vi "satellite simulator control.vi"() -> ()   [LabVIEW 2012]
uses:
  <vilib>/Utility/error.llb/DialogType.ctl
  <vilib>/DAQmx/create/channels.llb/DAQmx Create Channel (DO-Digital Output).vi
  <vilib>/Instr/_visa.llb/VISA Configure Serial Port (Instr).vi
  <vilib>/vision/NI_Vision_Development_Module.lvlib
  <vilib>/ptbypt/NI_PtbyPt.lvlib
panel:
  in  "Reaction Wheel":bool
  out "Write String":string
  in  "Control Value":sgl=1.5 format="%.4f"
  in  "Control Mode":u16(ring) items=["Idle"=0, "PWM (-1..1)"=1, "Current (-2.5..2.5A)"=2, "Speed (Rads/s)"=3, "Acceleration (Rads/sec^2)"=16, "Momentum (N-m-sec)"=17, "Torque (N-m)"=18]
  in  "Address":i32=11
  in  "Dst":i32=36
  in  "stop bits":u16(ring)=10 items=["1.0"=10, "1.5"=15, "2.0"=20]
  in  "VISA resource name (write)":refnum<visa-resource-name>="COM4"
  in  "flow control":u16(ring) items=["None"=0, "XON/XOFF"=1, "RTS/CTS"=2, "DTR/DSR"=4]
  in  "parity (0:none)":u16(ring) items=["None", "Odd", "Even", "Mark", "Space"]
  in  "data bits (8)":u16=8 min=5 max=8 step=1
  in  "baud rate (115200)":u32=115200
  out "bytes written":u32
  in  "bytes to read":u32=5
  out "Read string":string
  out "bytes read":u32
  out "Filtered Ohmega":dbl format="%0.2f"
  in  "VISA resource name":refnum<visa-resource-name>
  out "read buffer":string
  out "Ohmega":dbl[](graph)
  out "Filtered Ohmega":dbl[](graph)
  in  "Floating":bool
  in  "Thruster 8":bool
  in  "Thruster 7":bool
  in  "Thruster 6":bool
  in  "Thruster 5":bool
  in  "Thruster 4":bool
  in  "Thruster 3":bool
  in  "Thruster 2":bool
  in  "Truster1":bool
  in  "Thrusters Bundled":bool=TRUE
  in  "Manual Control Mode (Default)":bool
  in  "Up":bool
  in  "Right":bool
  in  "Down":bool
  in  "Left":bool
  in  "Stop 2":bool
  in  "CntrClk":bool
  in  "ClkWise":bool
  in  "Angular Acceleration":u16(ring) items=["Fast", "Slow"]
  in  "Duty Cycle":dbl=1.0
  in  "Automatic PD Position Controller":bool
  in  "Pixel-Distance Ratio (pix/cm)":dbl=8.26
  in  "Remote Logger Status":bool
  in  "Downlink Object Data?":bool
  in  "Remote Port":u16=61557
  in  "Local Port":u16=61556
  in  "Remote Host":string="localhost"
  in  "broadcast":bool
  in  "Maintain Attitude":bool
  out "alpha":dbl
  out "Objects":T1(array[cluster]) {"Aspect Ratio" format="%.2f"; "Orientation" format="%.2f"; "Area" format="%.2f"; "Object Center"."Y" format="%.2f"; "Object Center"."X" format="%.2f"}
  in  "Y Center Correction":dbl
  in  "X Center Correction":dbl
  out "Offset Degree":dbl
  in  "Y Desired":dbl
  in  "X Desired":dbl
  out "Vx (cm/s)":dbl
  out "Vy (cm/s)":dbl
  in  "OK Button":bool
  in  "Air Floating Status":bool
  in  "Control Freq":u32=20
  in  "Alpha Desired":dbl
  in  "STOP":bool caption="stop (F)"
  out "Image Out":T2(plugin-control)
  out "alpha (deg)":dbl
  out "dx (cm)":dbl
  out "dy (cm)":dbl
  # "Bundled Operations"
  # "Unbundled Operations"
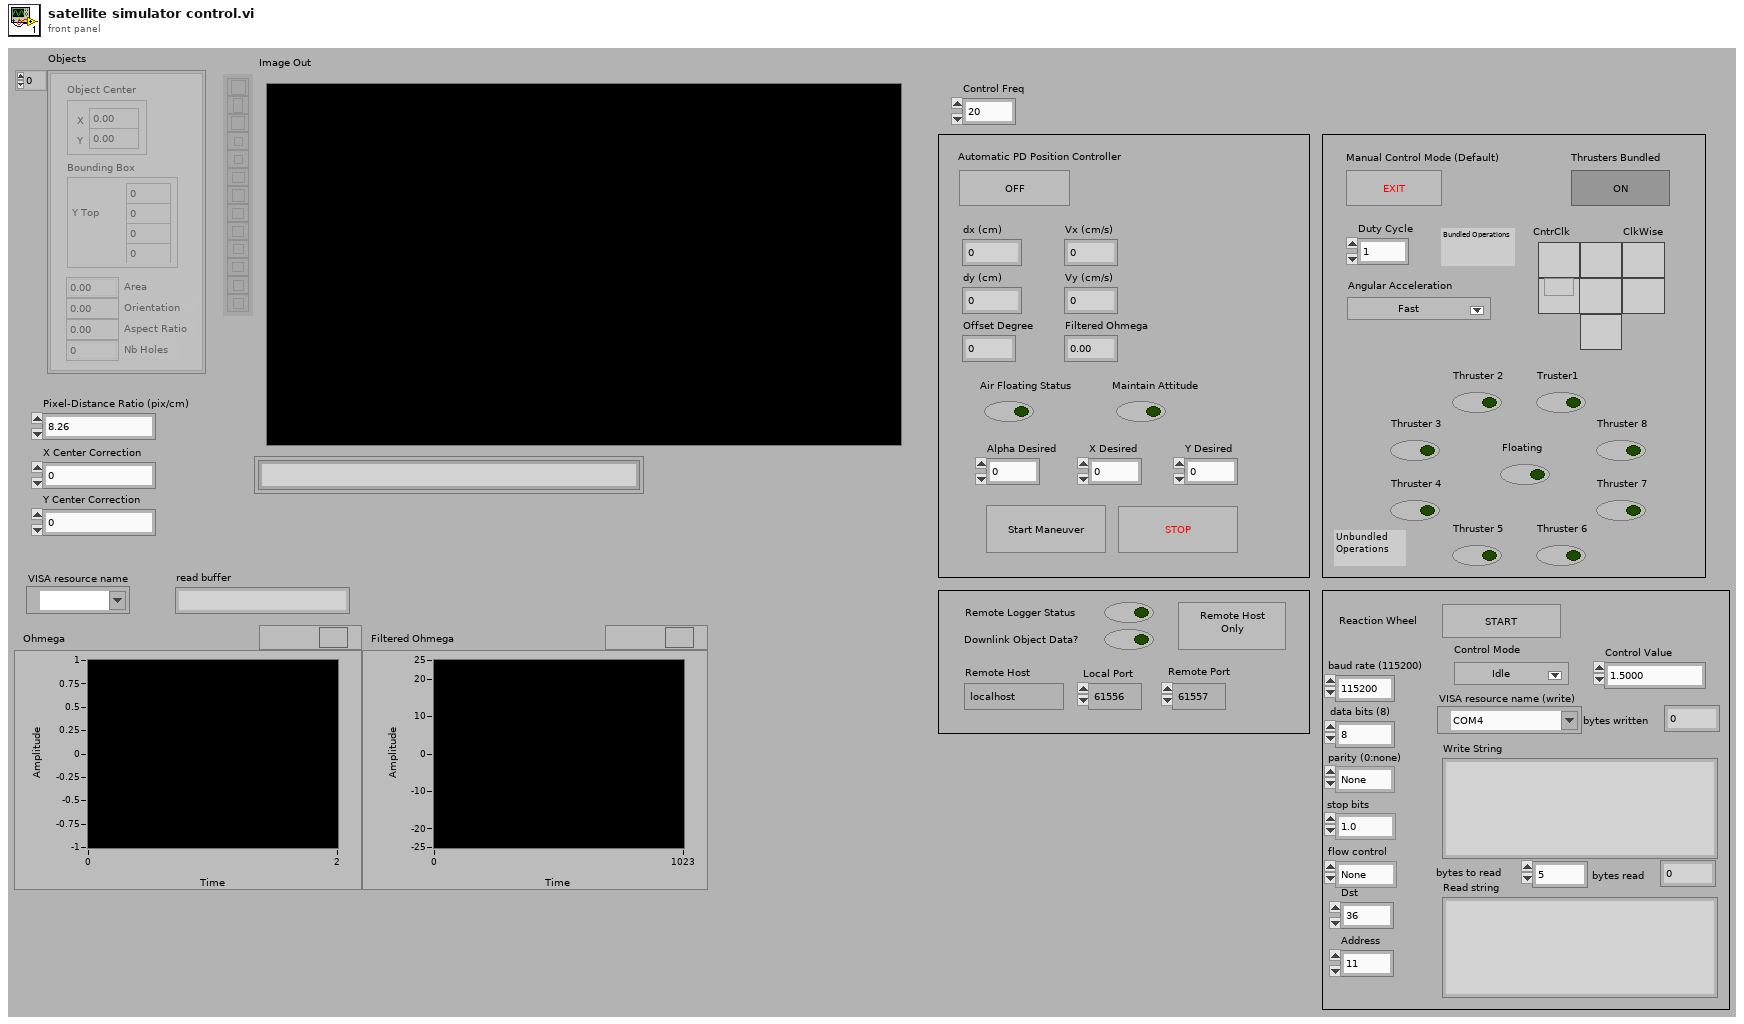
[diagram p1: front panel]
types:
  T1 = cluster{"Object Center":cluster{"X":sgl, "Y":sgl}, "Bounding Box":cluster{"X Left":i32, "Y Top":i32, "X Right":i32, "Y Bottom":i32}, "Area":sgl, "Orientation":sgl, "Aspect Ratio":sgl, "Nb Holes":i32}[]
  T2 = typedef "IMAQ Image.ctl" = refnum<image>
  T3 = typedef "DialogType.ctl" = u16
  T4 = cluster{"dx (cm)":dbl, "dy (cm)":dbl, "Offset Degree":dbl}
  T5 = cluster{"Objects":u16, "Threshold":i32, "Reject Border":bool, "Fill Holes":bool, "Min Object Size":bool, "Min Size":i32, "Max Object Size":bool, "Max Size":i32, "Show Search Area":bool, "Show Center":bool, "Show Bounding Box":bool}
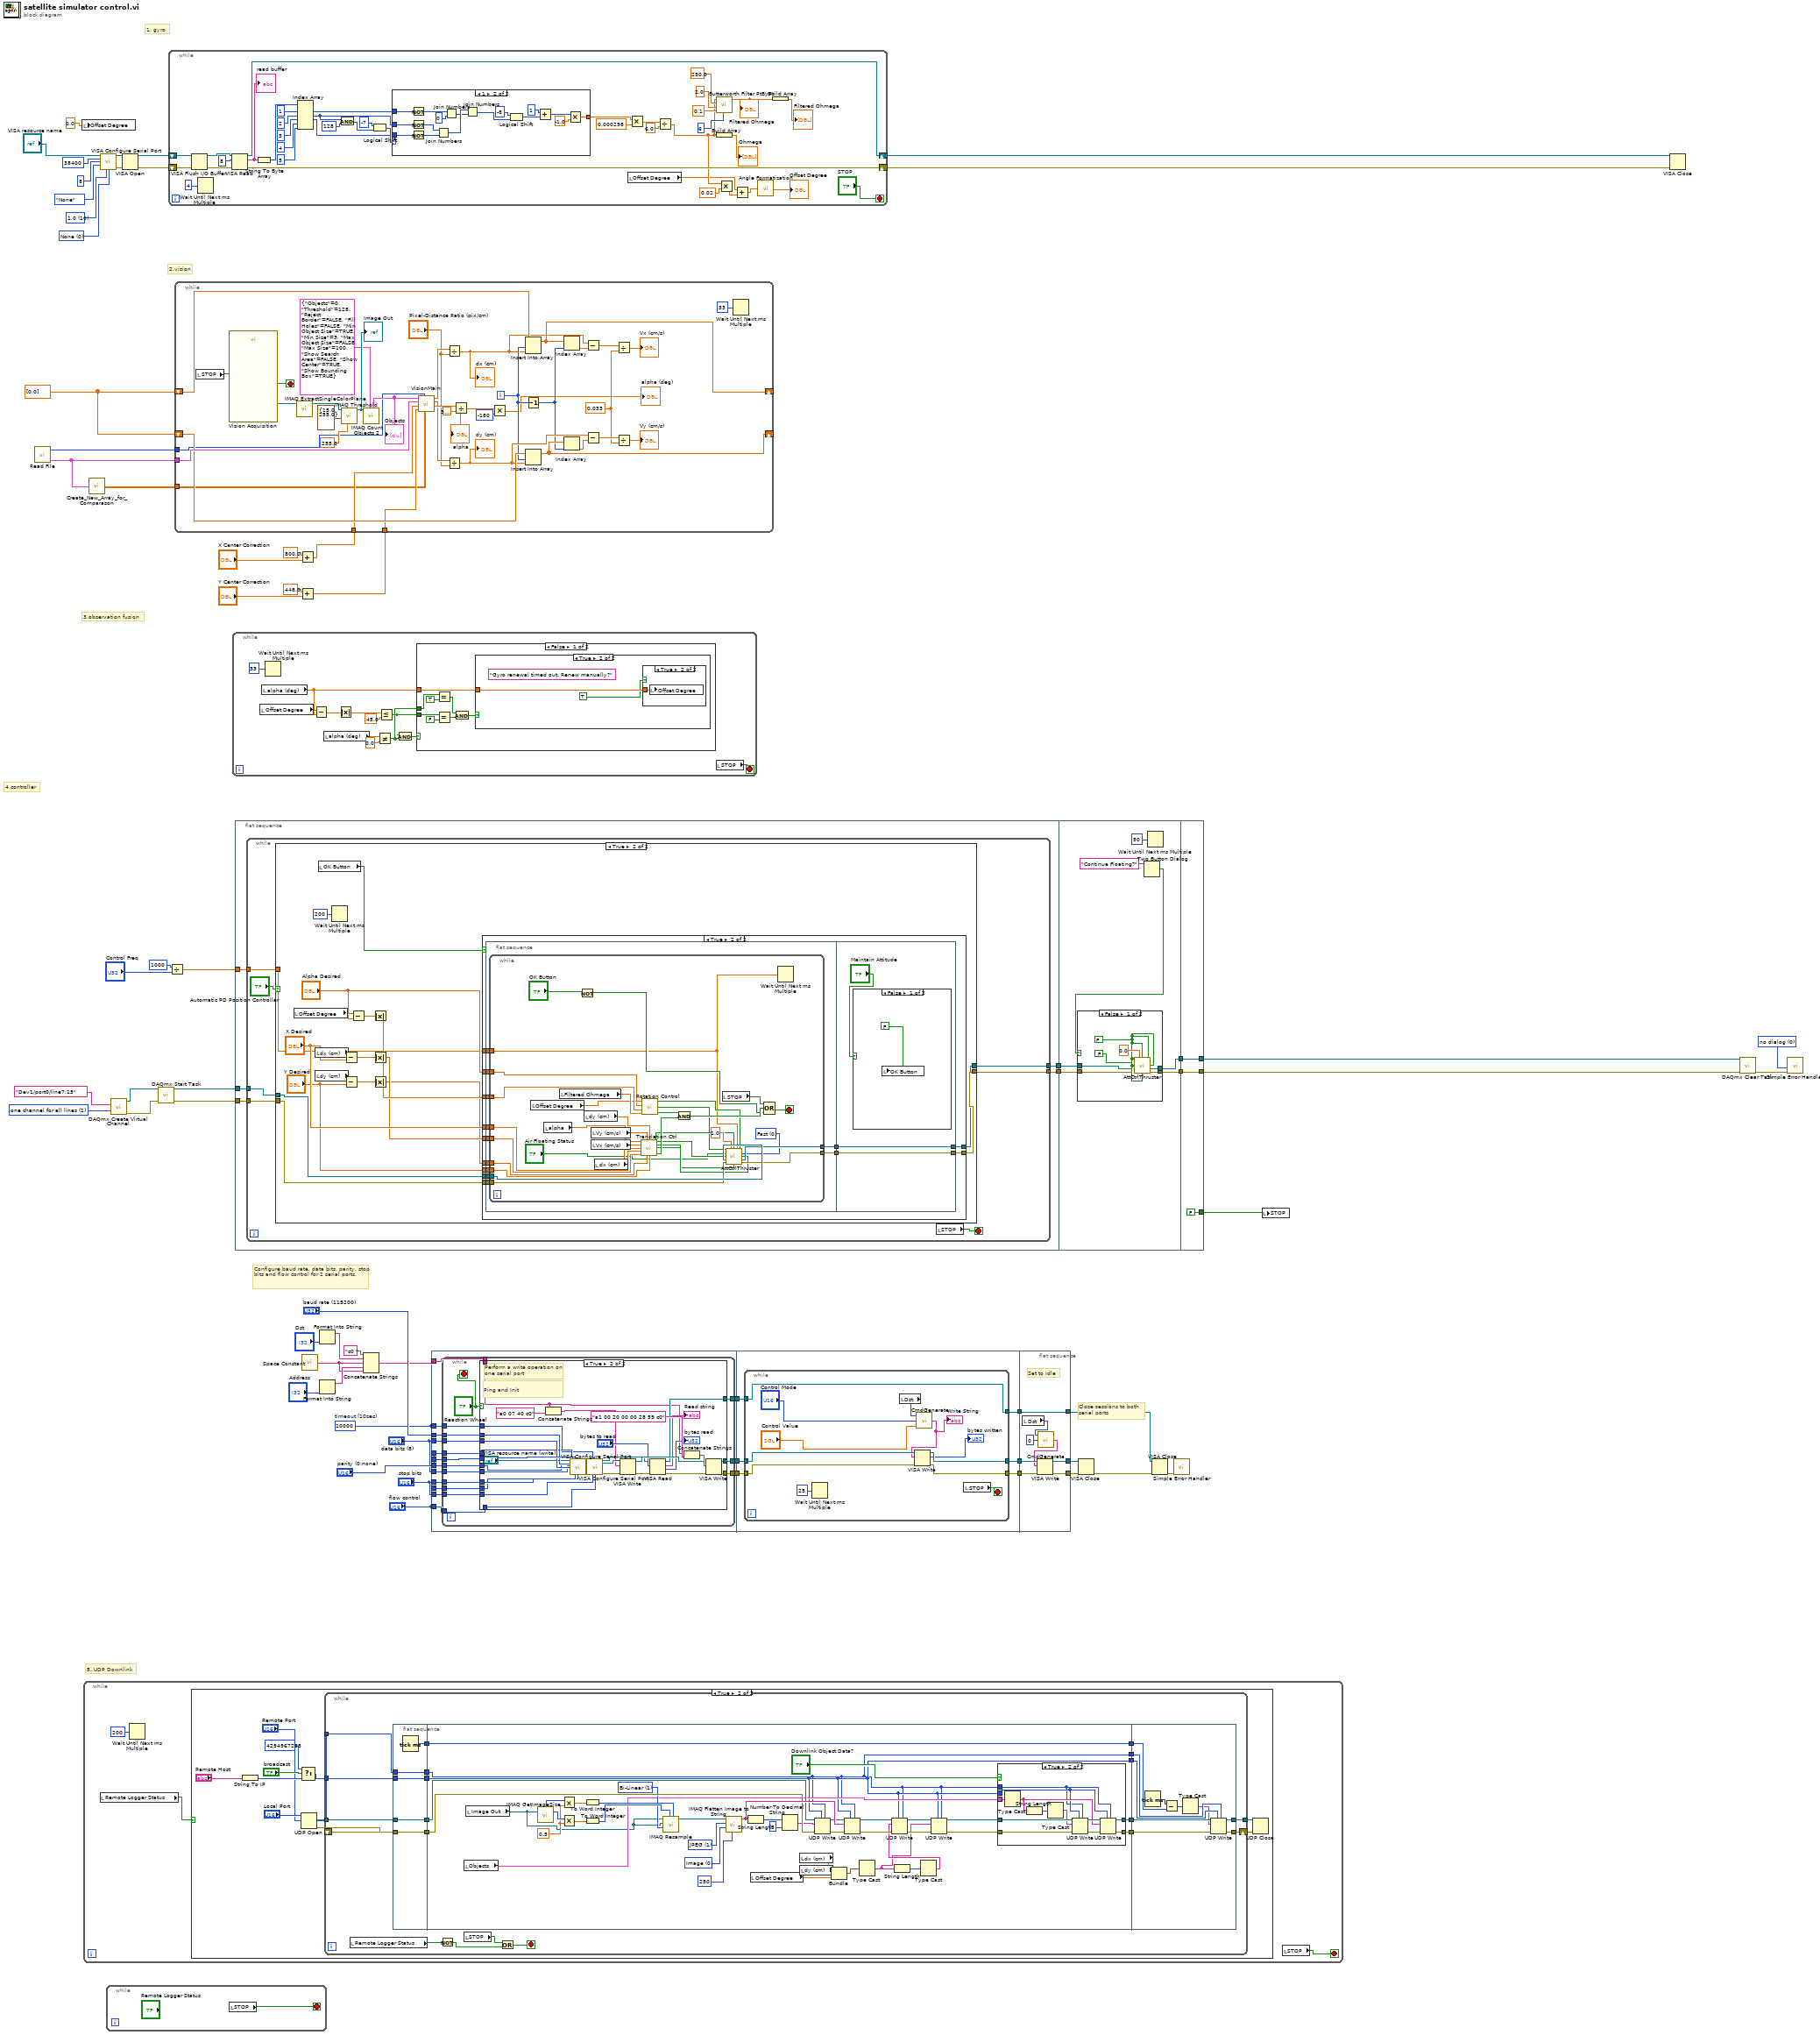
[diagram p0: block diagram]
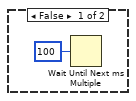
[diagram p2: hidden frame]
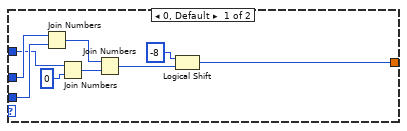
[diagram p3: hidden frame]
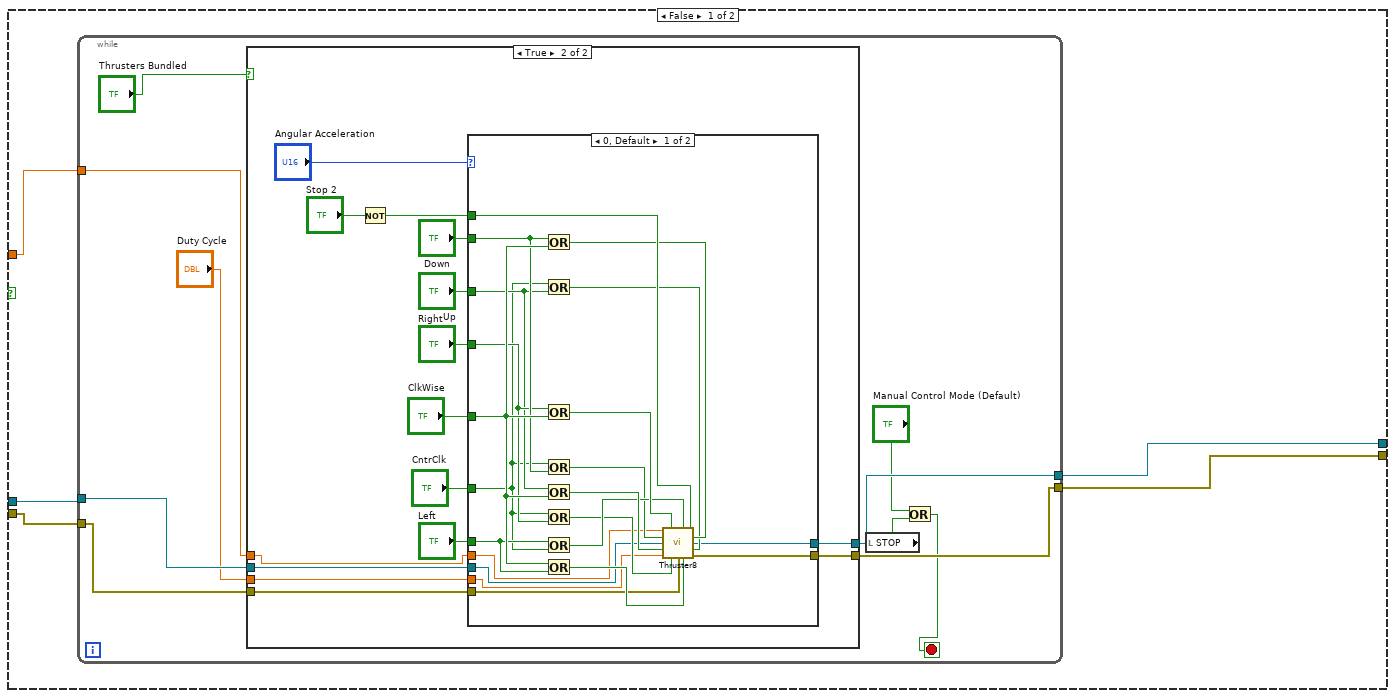
[diagram p6: hidden frame]
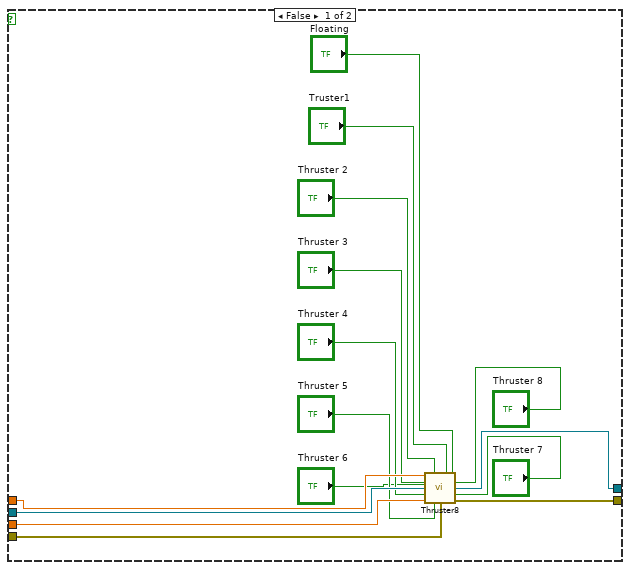
[diagram p7: hidden frame]
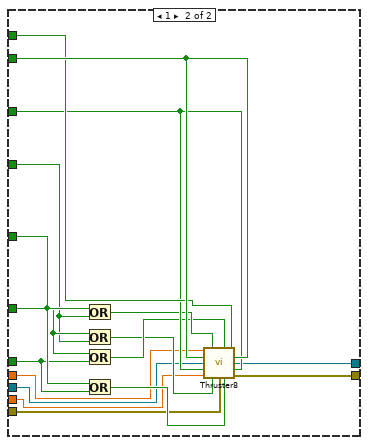
[diagram p8: hidden frame]
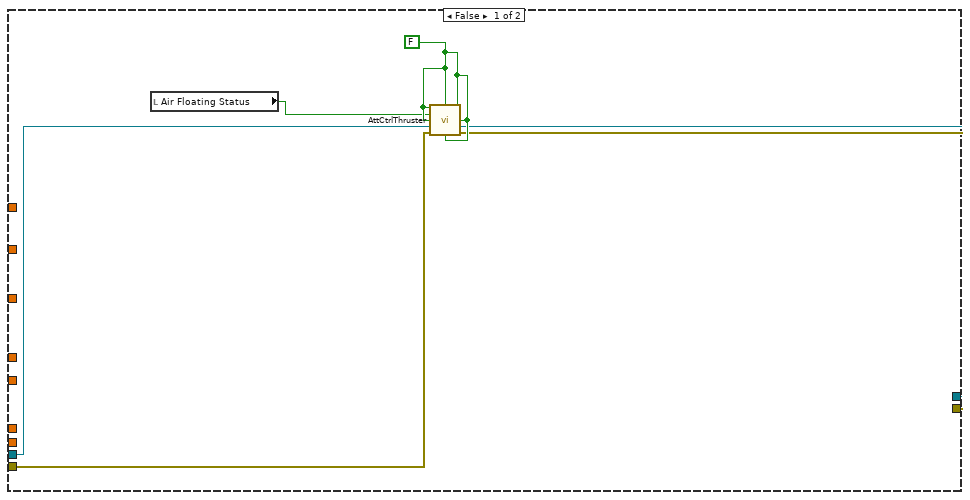
[diagram p9: hidden frame]
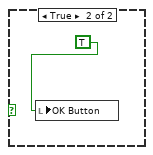
[diagram p10: hidden frame]
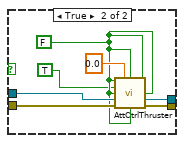
[diagram p11: hidden frame]
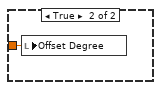
[diagram p14: hidden frame]
diagram:
  w11 = u32 10000  # timeout (10sec)
  w28 = u16 0 items=["None", "XON/XOFF", "RTS/CTS", "XON/XOFF & RTS/CTS", "DTR/DSR", "XON/XOFF & DTR/DSR"] ("flow control (0:none)")
  w30 = u16 10 items=["1.0"=10, "1.5"=15, "2.0"=20] ("stop bits (10: 1 bit)")
  w60 = T3 0 items=["no dialog", "OK message", "continue or stop message", "OK message + warnings", "continue/stop + warnings"] ("type of dialog (OK msg:1)")
  w63 = 1 items=["one channel for each line", "one channel for all lines"] ("line grouping")
  w49 = dbl[] [0.0]
  # "Close sessions to both serial ports"
  # "Configure baud rate, data bits, parity, stop bits and flow control for 2 serial ports."
  # "5. UDP Downlink"
  # "4.controller"
  # "3.observation fusion"
  # "2.vision"
  # "1. gyro"
  n1 = call "Read File.vi"() -> ("Objects"=w27:T1, "Total Obj"=w25:i32)  [unwired: 1 in]
  n2 = local write "Offset Degree"(0.0 ("y")) -> ()
  n3 = while {
    stop <- w67 stop-if-true
    n4 = local read "Remote Logger Status"() -> (w68:bool)
    n5 = Wait Until Next ms Multiple(millisecond multiple=u32 200) -> ()  [unwired: 1 out]
    n6 = case shown="True" w68 {
      frame False {
      }
      frame True {
        n7 = String To IP(1:"Remote Host") -> (0:w76:u32)
        n8 = Select(t=u32 4294967295, s="broadcast", f=w76) -> (s? t:f=w73:u32)
        n9 = UDP Open(11:"Local Port") -> (port=w72:refnum<k16>, 0:w71:errorcluster)  [unwired: 1 in, 4 out]
        n10 = while {
          tunnel: "Remote Port" -> [w99]
          tunnel: w73 -> [w98]
          tunnel: w72 -> [w97]
          tunnel: [w95] -> w70
          shift-right: [w94] -> w69
          shift-left: w71 -> [w96]
          stop <- w83 stop-if-true
          n11 = local read "Remote Logger Status"() -> (w81:bool)
          n12 = flat-sequence {
            tunnel: w97 -> [w101]
            tunnel: w99 -> [w102]
            tunnel: w98 -> [w103]
            tunnel: w96 -> [w104]
            tunnel: [w104] -> w93
            tunnel: [w103] -> w92
            tunnel: [w102] -> w91
            tunnel: [w101] -> w90
            tunnel: [w100] -> w89
            tunnel: [w124] -> w88
            tunnel: [w123] -> w87
            tunnel: w93 -> [w142]
            tunnel: w92 -> [w106]
            tunnel: w91 -> [w105]
            tunnel: w90 -> [w126]
            tunnel: [w125] -> w86
            tunnel: w89 -> [w125]
            tunnel: [w105] -> w85
            tunnel: [w106] -> w84
            tunnel: [w166] -> w95
            tunnel: [w160] -> w94
            tunnel: w88 -> [w161]
            tunnel: w87 -> [w167]
            tunnel: w86 -> [w168]
            tunnel: w85 -> [w165]
            tunnel: w84 -> [w164]
            frame #0 {
              n13 = Tick Count (ms)() -> (millisecond timer value=w100:u32)
            }
            frame #1 {
              w130 = u32 1 items=["Zero Order", "Bi-Linear", "Quadratic", "Cubic Spline"] ("Interpolation Type")
              w131 = 0.5
              w139 = 0 items=["Image", "Image and Vision Info", "Reference to Image"] ("Type of Flatten (Image and Vision Info)")
              w144 = 1 items=["None", "JPEG", "PACKED BINARY"] ("Compression (None)")
              n14 = local read "Objects"() -> (w121:T1)
              n15 = local read "Image Out"() -> (w120:T2)
              n16 = call "IMAQ GetImageSize"("Image"=w120) -> ("Y Resolution"=w132:i32, "X Resolution"=w133:i32)  [unwired: 3 in, 1 out]
              n17 = Multiply(x=w133, y=w131) -> (x*y=w135:dbl)
              n18 = Multiply(x=w132, y=w131) -> (x*y=w137:dbl)
              n19 = To Word Integer(number=w135) -> (16bit integer=w134:i16)
              n20 = To Word Integer(number=w137) -> (16bit integer=w136:i16)
              n21 = call "IMAQ Resample"("X Resolution"=w134, "Y Resolution"=w136, "Interpolation Type"=w130, "Image Dst"=w120, "Image Src"=w120) -> ("Image Dst Out"=w138:T2)  [unwired: 5 in, 1 out]
              n22 = call "IMAQ Flatten Image to String"("Quality (750)"=250, "Type of Flatten (Image and Vision Info)"=w139, "Compression (None)"=w144, "Image"=w138) -> ("Data String"=w143:string)  [unwired: 6 in, 1 out]
              n23 = String Length(string=w143) -> (length=w129:i32)
              n24 = local read "Offset Degree"() -> (w117:dbl)
              n25 = Number To Decimal String(number=w129, width (-)=i16 5) -> (decimal integer string=w128:string)
              n26 = local read "dx (cm)"() -> (w119:dbl)
              n27 = local read "dy (cm)"() -> (w118:dbl)
              n28 = UDP Write(address=w106, port or service name=w105, connection ID=w126, data in=w128, 8:w142) -> (error out=w141:errorcluster, 3:w140:refnum<k16>)  [unwired: 1 out]
              n29 = Bundle("dx (cm)"=w119, "dy (cm)"=w118, "Offset Degree"=w117) -> (w116:T4)  [unwired: 1 in]
              n30 = UDP Write(address=w106, port or service name=w105, connection ID=w140, data in=w143, 8:w141) -> (error out=w114:errorcluster, 3:w115:refnum<k16>)  [unwired: 1 out]
              n31 = Type Cast(x=w116) -> (*(type *) &x=w107:string)  [unwired: 1 in]
              n32 = String Length(string=w107) -> (length=w109:i32)
              n33 = Type Cast(x=w109) -> (*(type *) &x=w108:string)  [unwired: 1 in]
              n34 = UDP Write(address=w106, port or service name=w105, connection ID=w115, data in=w108, 8:w114) -> (error out=w113:errorcluster, 3:w111:refnum<k16>)  [unwired: 1 out]
              n35 = UDP Write(address=w106, port or service name=w105, connection ID=w111, data in=w107, 8:w113) -> (error out=w112:errorcluster, 3:w110:refnum<k16>)  [unwired: 1 out]
              n36 = case shown="True" "Downlink Object Data?" {
                tunnel: w121 -> [_ w159]
                tunnel: w112 -> [w147 w157]
                tunnel: [w147 w155] -> w124
                tunnel: w110 -> [w146 w154]
                tunnel: [w146 w152] -> w123
                tunnel: w106 -> [_ w149]
                tunnel: w105 -> [_ w148]
                frame False {
                }
                frame True {
                  n37 = Type Cast(x=w159) -> (*(type *) &x=w150:string)  [unwired: 1 in]
                  n38 = String Length(string=w150) -> (length=w158:i32)
                  n39 = Type Cast(x=w158) -> (*(type *) &x=w151:string)  [unwired: 1 in]
                  n40 = UDP Write(address=w149, port or service name=w148, connection ID=w154, data in=w151, 8:w157) -> (error out=w156:errorcluster, 3:w153:refnum<k16>)  [unwired: 1 out]
                  n41 = UDP Write(address=w149, port or service name=w148, connection ID=w153, data in=w150, 8:w156) -> (error out=w155:errorcluster, 3:w152:refnum<k16>)  [unwired: 1 out]
                }
              }
            }
            frame #2 {
              n42 = Tick Count (ms)() -> (millisecond timer value=w169:u32)
              n43 = Subtract(x=w169, y=w168) -> (x-y=w163:u32)
              n44 = Type Cast(x=w163) -> (*(type *) &x=w162:string)  [unwired: 1 in]
              n45 = UDP Write(address=w164, port or service name=w165, connection ID=w167, data in=w162, 8:w161) -> (error out=w160:errorcluster, 3:w166:refnum<k16>)  [unwired: 1 out]
            }
          }
          n46 = Not(x=w81) -> (.not. x?=w80:bool)
          n47 = local read "STOP"() -> (w82:bool)
          n48 = Or(x=w82, y=w80) -> (x .or. y?=w83:bool)
        }
        n49 = UDP Close(connection ID=w70, 8:w69) -> ()  [unwired: 2 out]
      }
    }
    n50 = local read "STOP"() -> (w67:bool)
  }
  n51 = call "Create_New_Array_for_Comparason.vi"("Captured Plots"=w27) -> ("Generated Distance Array"=w26:dbl[][])
  n52 = call-poly "VISA Configure Serial Port"("VISA resource name"="VISA resource name", "baud rate (9600)"=u32 38400, "data bits (8)"=u16 8, "parity (0:none)"=enum16{"None", "Odd", "Even", "Mark", "Space"}."None", "stop bits (10: 1 bit)"=w30, "flow control (0:none)"=w28) -> ("VISA resource name out"=w37:refnum<visa-resource-name>, "error out"=w36:errorcluster)  [unwired: 8 in]
  n53 = while {
    stop <- w170 stop-if-true
    n54 = local read "STOP"() -> (w170:bool)
  }
  n55 = call-poly <vilib>:"DAQmx Create Virtual Channel.vi"("lines"=tag "Dev1/port0/line7:15" ("Lines"), "line grouping"=w63) -> ("task out"=w61:refnum<k21>, "error out"=w62:errorcluster)  [unwired: 12 in]
  n56 = VISA Open(error in (no error)=w36, VISA resource name=w37) -> (VISA resource name=w35:refnum<visa-resource-name>, error out=w34:errorcluster)  [unwired: 3 in]
  n57 = call <vilib>:"DAQmx Start Task.vi"("task/channels in"=w61, "error in"=w62) -> ("task out"=w56:refnum<k21>, "error out"=w55:errorcluster)  [unwired: 12 in]
  n58 = while {
    shift-right: [w178] -> w32
    shift-left: w34 -> [w208]
    shift-right: [w179] -> w33
    shift-left: w35 -> [w209]
    stop <- "STOP" stop-if-true
    n59 = VISA Flush I/O Buffer(VISA resource name=w209, error in (no error)=w208) -> (VISA resource name out=w207:refnum<visa-resource-name>, error out=w206:errorcluster)  [unwired: 1 in]
    n60 = Wait Until Next ms Multiple(millisecond multiple=u32 4) -> ()  [unwired: 1 out]
    n61 = VISA Read(VISA resource name=w207, byte count=u32 8, error in (no error)=w206) -> (VISA resource name out=w179:refnum<visa-resource-name>, read buffer=w180:string, error out=w178:errorcluster)  [unwired: 1 out]
    "read buffer" <- w180
    n62 = String To Byte Array(string=w180) -> (unsigned byte array=w201:u8[])
    n63 = Index Array(array=w201, index #1=1 ("index"), index #2=2 ("index"), index #3=3 ("index"), index #4=4 ("index"), index #5=5 ("index")) -> (element #1=w185:u8, element #2=w184:u8, element #3=w183:u8)  [unwired: 2 out]
    n64 = And(x=w184, y=u8 128) -> (x .and. y?=w195:u8)
    n65 = Logical Shift(y=i16 -7, x=w195) -> (x << y=w193:u8)
    n66 = case shown="1" w193 {
      tunnel: [w211 w220] -> w197
      tunnel: w185 -> [w212 w230]
      tunnel: w184 -> [w214 w229]
      tunnel: w183 -> [w213 w228]
      frame 0, Default {
        n67 = Join Numbers(hi=w214, lo=w213) -> ((hi.lo)=w219:u16)
        n68 = Join Numbers(hi=w212, lo=u8 0) -> ((hi.lo)=w217:u16)
        n69 = Join Numbers(hi=w219, lo=w217) -> ((hi.lo)=w216:u32)
        n70 = Logical Shift(y=i16 -8, x=w216) -> (x << y=w211:u32)
      }
      frame 1 {
        n71 = Not(x=w230) -> (.not. x?=w225:u8)
        n72 = Not(x=w229) -> (.not. x?=w227:u8)
        n73 = Not(x=w228) -> (.not. x?=w226:u8)
        n74 = Join Numbers(hi=w227, lo=w226) -> ((hi.lo)=w235:u16)
        n75 = Join Numbers(hi=w225, lo=u8 0) -> ((hi.lo)=w233:u16)
        n76 = Join Numbers(hi=w235, lo=w233) -> ((hi.lo)=w232:u32)
        n77 = Logical Shift(y=i16 -8, x=w232) -> (x << y=w224:u32)
        n78 = Add(x=u32 1, y=w224) -> (x+y=w221:u32)
        n79 = Multiply(x=w221, y=-1.0) -> (x*y=w220:dbl)
      }
    }
    n80 = local read "Offset Degree"() -> (w174:dbl)
    n81 = Multiply(x=w197, y=0.000298) -> (x*y=w203:dbl)
    n82 = Divide(x=w203, y=6.0) -> (x/y=w175:dbl)
    n83 = call <vilib>:"Butterworth Filter PtByPt.vi"("order"=6, "low cutoff freq: fl"=0.1, "high cutoff freq: fh"=2.0, "sampling freq: fs"=250.0, "x"=w175) -> ("Filtered x"=w187:dbl)  [unwired: 4 in, 1 out]
    "Filtered Ohmega" <- w187
    n84 = Build Array(w175) -> (→"Ohmega":dbl[])
    n85 = Multiply(x=w175, y=0.02) -> (x*y=w173:dbl)
    n86 = Add(x=w174, y=w173) -> (x+y=w172:dbl)
    n87 = call "Angle Formatization.vi"("Alpha"=w172) -> ("Alpha Formatized"=→"Offset Degree":dbl)
    n88 = Build Array(w187) -> (→"Filtered Ohmega":dbl[])
  }
  n89 = Divide(x=u32 1000 ("milliseconds to wait"), y="Control Freq") -> (x/y=w52:dbl)
  n90 = while {
    stop <- w246 stop-if-true
    n91 = local read "Offset Degree"() -> (w245:dbl)
    n92 = local read "alpha (deg)"() -> (w241:dbl)
    n93 = Wait Until Next ms Multiple(millisecond multiple=u32 33) -> ()  [unwired: 1 out]
    n94 = Subtract(x=w245, y=w241) -> (x-y=w244:dbl)
    n95 = local read "alpha (deg)"() -> (w239:dbl)
    n96 = Absolute Value(x=w244) -> (abs(x)=w243:dbl)
    n97 = Not Equal?(x=w239, y=0.0) -> (x != y?=w237:bool)
    n98 = Less Or Equal?(x=w243, y=45.0) -> (x <= y?=w236:bool)
    n99 = And(x=w236, y=w237) -> (x .and. y?=w240:bool)
    n100 = case shown="False" w240 {
      tunnel: w241 -> [w248 w259]
      tunnel: w237 -> [w250 _]
      tunnel: w236 -> [w249 _]
      frame False {
        n101 = Equal?(x=w250, y=TRUE) -> (x = y?=w254:bool)
        n102 = Equal?(x=w249, y=FALSE) -> (x = y?=w253:bool)
        n103 = And(x=w254, y=w253) -> (x .and. y?=w251:bool)
        n104 = case shown="True" w251 {
          tunnel: w248 -> [_ w257]
          frame False {
          }
          frame True {
            (unwired) "Gyro renewal timed out. Renew manually?" ("message")
            n105 = case shown="True" TRUE {
              tunnel: w257 -> [_ w258]
              frame False {
              }
              frame True {
                n106 = local write "Offset Degree"(w258) -> ()
              }
            }
          }
        }
      }
      frame True {
        n107 = local write "Offset Degree"(w259) -> ()
      }
    }
    n108 = local read "STOP"() -> (w246:bool)
  }
  n109 = flat-sequence {
    tunnel: w56 -> [w264]
    tunnel: w55 -> [w263]
    tunnel: w52 -> [w260]
    tunnel: [w262] -> w51
    tunnel: [w261] -> w50
    tunnel: w51 -> [w449]
    tunnel: w50 -> [w447]
    tunnel: [w448] -> w42
    tunnel: [w446] -> w41
    tunnel: [w465] -> w53
    tunnel: [w466] -> w54
    tunnel: w42 -> [w466]
    tunnel: w41 -> [w465]
    tunnel: [FALSE] -> w40
    frame #0 {
      n110 = while {
        tunnel: w264 -> [w271]
        tunnel: w263 -> [w270]
        tunnel: [w269] -> w262
        tunnel: [w268] -> w261
        tunnel: w260 -> [w266]
        stop <- w267 stop-if-true
        n111 = case shown="True" "Automatic PD Position Controller" {
          tunnel: w271 -> [w275 w373]
          tunnel: w270 -> [w274 w372]
          tunnel: [w272 w371] -> w269
          tunnel: [w273 w370] -> w268
          tunnel: w266 -> [w276 w356]
          frame False {
            n112 = while {
              tunnel: w276 -> [w286]
              tunnel: w275 -> [w285]
              tunnel: [w284] -> w273
              tunnel: [w283] -> w272
              tunnel: w274 -> [w282]
              stop <- w279 stop-if-true
              n113 = case shown="True" "Thrusters Bundled" {
                tunnel: w286 -> [w297 w309]
                tunnel: w285 -> [w301 w308]
                tunnel: [w298 w307] -> w284
                tunnel: [w299 w306] -> w283
                tunnel: w282 -> [w300 w305]
                tunnel: "Duty Cycle" -> [w296 w302]
                frame False {
                  n114 = call "Thruster8.vi"("period"=w297, "Thruster 2"="Thruster 2", "Truster1"="Truster1", "Floating"="Floating", "Thruster 3"="Thruster 3", "Thruster 8"="Thruster 8", "task in"=w301, "Thruster 4"="Thruster 4", "Thruster 7"="Thruster 7", "Duty Cycle"=w296, "Thruster 5"="Thruster 5", "error in"=w300, "Thruster 6"="Thruster 6") -> ("task out"=w298:refnum<k21>, "error out"=w299:errorcluster)  [unwired: 1 in]
                }
                frame True {
                  n115 = Not(x="Stop 2") -> (.not. x?=w303:bool)
                  n116 = case shown="0, Default" "Angular Acceleration" {
                    tunnel: w303 -> [w337 w353]
                    tunnel: "Down" -> [w329 w354]
                    tunnel: "Left" -> [w331 w347]
                    tunnel: "Up" -> [w325 w352]
                    tunnel: "Right" -> [w327 w345]
                    tunnel: "ClkWise" -> [w333 w351]
                    tunnel: "CntrClk" -> [w324 w348]
                    tunnel: w302 -> [w322 w343]
                    tunnel: w309 -> [w321 w342]
                    tunnel: w308 -> [w320 w338]
                    tunnel: [w319 w339] -> w307
                    tunnel: [w318 w340] -> w306
                    tunnel: w305 -> [w317 w341]
                    frame 0, Default {
                      n117 = Or(x=w329, y=w333) -> (x .or. y?=w332:bool)
                      n118 = Or(x=w324, y=w325) -> (x .or. y?=w323:bool)
                      n119 = Or(x=w327, y=w333) -> (x .or. y?=w335:bool)
                      n120 = Or(x=w324, y=w329) -> (x .or. y?=w328:bool)
                      n121 = Or(x=w325, y=w333) -> (x .or. y?=w336:bool)
                      n122 = Or(x=w324, y=w327) -> (x .or. y?=w326:bool)
                      n123 = Or(x=w331, y=w324) -> (x .or. y?=w330:bool)
                      n124 = Or(x=w333, y=w331) -> (x .or. y?=w334:bool)
                      n125 = call "Thruster8.vi"("period"=w321, "Thruster 2"=w335, "Truster1"=w330, "Floating"=w337, "Thruster 3"=w328, "Thruster 8"=w332, "task in"=w320, "Thruster 4"=w336, "Thruster 7"=w323, "Duty Cycle"=w322, "Thruster 5"=w326, "error in"=w317, "Thruster 6"=w334) -> ("task out"=w319:refnum<k21>, "error out"=w318:errorcluster)  [unwired: 1 in]
                    }
                    frame 1 {
                      n126 = Or(x=w351, y=w345) -> (x .or. y?=w350:bool)
                      n127 = Or(x=w348, y=w345) -> (x .or. y?=w344:bool)
                      n128 = Or(x=w348, y=w347) -> (x .or. y?=w346:bool)
                      n129 = Or(x=w351, y=w347) -> (x .or. y?=w349:bool)
                      n130 = call "Thruster8.vi"("period"=w342, "Thruster 2"=w350, "Truster1"=w346, "Floating"=w353, "Thruster 3"=w354, "Thruster 8"=w354, "task in"=w338, "Thruster 4"=w352, "Thruster 7"=w352, "Duty Cycle"=w343, "Thruster 5"=w344, "error in"=w341, "Thruster 6"=w349) -> ("task out"=w339:refnum<k21>, "error out"=w340:errorcluster)  [unwired: 1 in]
                    }
                  }
                }
              }
              n131 = local read "STOP"() -> (w281:bool)
              n132 = Or(x="Manual Control Mode (Default)", y=w281) -> (x .or. y?=w279:bool)
            }
          }
          frame True {
            n133 = local read "Offset Degree"() -> (w369:dbl)
            n134 = local read "dx (cm)"() -> (w365:dbl)
            n135 = local read "dy (cm)"() -> (w361:dbl)
            n136 = local read "OK Button"() -> (w357:bool)
            n137 = Wait Until Next ms Multiple(millisecond multiple=u32 200) -> ()  [unwired: 1 out]
            n138 = Subtract(x=w365, y="X Desired") -> (x-y=w363:dbl)
            n139 = Subtract(x=w361, y="Y Desired") -> (x-y=w359:dbl)
            n140 = Subtract(x=w369, y="Alpha Desired") -> (x-y=w367:dbl)
            n141 = Absolute Value(x=w367) -> (abs(x)=w366:dbl)
            n142 = Absolute Value(x=w363) -> (abs(x)=w362:dbl)
            n143 = Absolute Value(x=w359) -> (abs(x)=w358:dbl)
            n144 = case shown="True" w357 {
              tunnel: w373 -> [w377 w392]
              tunnel: w372 -> [w376 w391]
              tunnel: [w375 w390] -> w371
              tunnel: [w374 w389] -> w370
              tunnel: w356 -> [_ w388]
              tunnel: "Alpha Desired" -> [_ w387]
              tunnel: w366 -> [_ w386]
              tunnel: "X Desired" -> [_ w385]
              tunnel: w362 -> [_ w384]
              tunnel: "Y Desired" -> [_ w383]
              tunnel: w358 -> [_ w382]
              frame False {
                w379 = FALSE
                n145 = local read "Air Floating Status"() -> (w378:bool)
                n146 = call "AttCtrlThruster.vi"("ctclk"=w379, "Up"=w379, "clkwis"=w379, "Float"=w378, "Left"=w379, "Right"=w379, "task in"=w377, "error in"=w376, "Down"=w379) -> ("task out"=w374:refnum<k21>, "error out"=w375:errorcluster)  [unwired: 5 in]
              }
              frame True {
                n147 = flat-sequence {
                  tunnel: w392 -> [w403]
                  tunnel: w391 -> [w402]
                  tunnel: w388 -> [w399]
                  tunnel: w387 -> [w398]
                  tunnel: w386 -> [w397]
                  tunnel: w385 -> [w396]
                  tunnel: w384 -> [w395]
                  tunnel: w383 -> [w394]
                  tunnel: w382 -> [w393]
                  tunnel: [w401] -> w381
                  tunnel: [w400] -> w380
                  tunnel: [w439] -> w389
                  tunnel: [w440] -> w390
                  tunnel: w381 -> [w440]
                  tunnel: w380 -> [w439]
                  frame #0 {
                    n148 = while {
                      tunnel: w403 -> [w437]
                      tunnel: w402 -> [w436]
                      tunnel: [w434] -> w401
                      tunnel: [w435] -> w400
                      tunnel: w399 -> [w405]
                      tunnel: w398 -> [w415]
                      tunnel: w397 -> [w430]
                      tunnel: w396 -> [w414]
                      tunnel: w395 -> [w425]
                      tunnel: w394 -> [w413]
                      tunnel: w393 -> [w412]
                      stop <- w431 stop-if-true
                      w421 = u16 0 items=["Fast", "Slow"] ("Angular Acceleration")
                      n149 = local read "Offset Degree"() -> (w428:dbl)
                      n150 = local read "alpha"() -> (w409:dbl)
                      n151 = local read "Filtered Ohmega"() -> (w429:dbl)
                      n152 = Not(x="OK Button") -> (.not. x?=w410:bool)
                      n153 = local read "dy (cm)"() -> (w423:dbl)
                      n154 = local read "Vy (cm/s)"() -> (w424:dbl)
                      n155 = local read "Vx (cm/s)"() -> (w427:dbl)
                      n156 = local read "dx (cm)"() -> (w426:dbl)
                      n157 = call "Translation Ctrl.vi"("Alpha"=w409, "Filtered Speed Y"=w424, "Y In"=w423, "Filtered Speed X"=w427, "X In"=w426, "X Desired"=w414, "Original Difference X"=w425, "Original Difference Y"=w412, "Y Desired"=w413) -> ("Left"=w419:bool, "Right"=w418:bool, "Down"=w417:bool, "Up"=w416:bool, "Maneuver Complete?"=w420:bool)  [unwired: 2 in]
                      n158 = call "Rotation Control.vi"("Filtered Ohmega"=w429, "Original Difference"=w430, "Alpha Desired"=w415, "Alpha In"=w428) -> ("Maneuver Complete?"=w408:bool, "Counter-ClkWise Rot Ctrl"=w407:bool, "Clockwise Rot Ctrl"=w406:bool)
                      n159 = And(x=w408, y=w420) -> (x .and. y?=w422:bool)
                      n160 = local read "STOP"() -> (w432:bool)
                      n161 = call "AttCtrlThruster.vi"("ctclk"=w407, "Duty Cycle"=1.0, "Up"=w416, "Period"=w405, "clkwis"=w406, "Float"="Air Floating Status", "Angular Acceleration"=w421, "Left"=w419, "Right"=w418, "task in"=w437, "error in"=w436, "Down"=w417) -> ("task out"=w435:refnum<k21>, "error out"=w434:errorcluster)  [unwired: 2 in]
                      n162 = Compound Arithmetic op=OR(w432, w422, w410) -> (w431:bool)
                      n163 = Wait Until Next ms Multiple(millisecond multiple=w405) -> ()  [unwired: 1 out]
                    }
                  }
                  frame #1 {
                    n164 = case shown="False" "Maintain Attitude" {
                      frame False {
                        n165 = local write "OK Button"(FALSE) -> ()
                      }
                      frame True {
                        n166 = local write "OK Button"(TRUE) -> ()
                      }
                    }
                  }
                }
              }
            }
          }
        }
        n167 = local read "STOP"() -> (w267:bool)
      }
    }
    frame #1 {
      n168 = Two Button Dialog(message="Continue Floating?") -> (T button?=w443:bool)  [unwired: 2 in]
      n169 = case shown="False" w443 {
        tunnel: w449 -> [w452 w463]
        tunnel: [w450 w462] -> w448
        tunnel: w447 -> [w453 w461]
        tunnel: [w451 w460] -> w446
        frame False {
          w455 = FALSE
          n170 = call "AttCtrlThruster.vi"("ctclk"=w455, "Duty Cycle"=0.0, "Up"=w455, "clkwis"=w455, "Float"=FALSE, "Left"=w455, "Right"=w455, "task in"=w453, "error in"=w452, "Down"=w455) -> ("task out"=w451:refnum<k21>, "error out"=w450:errorcluster)  [unwired: 4 in]
        }
        frame True {
          w458 = FALSE
          n171 = call "AttCtrlThruster.vi"("ctclk"=w458, "Duty Cycle"=0.0, "Up"=w458, "clkwis"=w458, "Float"=TRUE, "Left"=w458, "Right"=w458, "task in"=w461, "error in"=w463, "Down"=w458) -> ("task out"=w460:refnum<k21>, "error out"=w462:errorcluster)  [unwired: 4 in]
        }
      }
      n172 = Wait Until Next ms Multiple(millisecond multiple=u32 50) -> ()  [unwired: 1 out]
    }
    frame #2 {
    }
  }
  n173 = Add(x=800.0 ("c_x"), y="X Center Correction") -> (x+y=w46:dbl)
  n174 = Add(x=448.0 ("c_y"), y="Y Center Correction") -> (x+y=w43:dbl)
  n175 = while {
    tunnel: w27 -> [w493]
    shift-right: [w490] -> _
    shift-left: w49 -> [w491]
    shift-right: [w479] -> _
    shift-left: w49 -> [w482]
    tunnel: w43 -> [w472]
    tunnel: w46 -> [w471]
    tunnel: w26 -> [w468]
    tunnel: w25 -> [w467]
    i -> [w481]
    stop <- w504 stop-if-true
    w475 = 0.033 ("y")
    n176 = local read "STOP"() -> (w495:bool)
    n177 = call "Vision Acquisition"("Stop (F)"=w495) -> ("Image Out"=w499:T2, "Stopped"=w504:bool)  [unwired: 24 in, 1 out]
    n178 = call "IMAQ ExtractSingleColorPlane"("Image Src"=w499) -> ("Image Dst Out"=w503:T2)  [unwired: 9 in, 1 out]
    n179 = call "IMAQ Threshold"("Replace Value"=sgl 255.0 ("replace value"), "Range"=cluster{"lower value":sgl, "upper value":sgl} {"lower value"=15.0, "upper value"=255.0} ("threshold"), "Image Src"=w503) -> ("Image Dst Out"=w500:T2)  [unwired: 7 in, 1 out]
    "Image Out" <- w500
    n180 = call "IMAQ Count Objects 2"("Settings"=T5 {"Objects"=0, "Threshold"=128, "Reject Border"=FALSE, "Fill Holes"=FALSE, "Min Object Size"=TRUE, "Min Size"=3, "Max Object Size"=FALSE, "Max Size"=100, "Show Search Area"=FALSE, "Show Center"=TRUE, "Show Bounding Box"=TRUE}, "Image"=w500) -> ("Objects"=w494:T1)  [unwired: 5 in, 4 out]
    "Objects" <- w494
    n181 = call "VisionMain.vi"("Generated Distance Array"=w468, "Database Total Points"=w467, "Y Center"=w472, "X Center"=w471, "Original Plots"=w493, "Plots Captured"=w494) -> ("alpha"=w492:dbl, "dy"=w488:dbl, "dx"=w483:dbl)  [unwired: 3 in]
    "alpha" <- w492
    n182 = Divide(x=w483, y="Pixel-Distance Ratio (pix/cm)") -> (x/y=w478:dbl)
    "dx (cm)" <- w478
    n183 = Divide(x=w488, y="Pixel-Distance Ratio (pix/cm)") -> (x/y=w487:dbl)
    "dy (cm)" <- w487
    n184 = Divide(x=w492, y=3.141592653589793) -> (x/y=w497:dbl)
    n185 = Multiply(x=w497, y=-180) -> (x*y=→"alpha (deg)":dbl)
    n186 = Insert Into Array(array=w482, index=w481, new element=w478) -> (w479:dbl[])
    n187 = Insert Into Array(array=w491, index=w481, new element=w487) -> (w490:dbl[])
    n188 = Decrement(x=w481) -> (x-1=w480:i32)
    n189 = Index Array(array=w479, index=w480) -> (element=w477:dbl)
    n190 = Index Array(array=w490, index=w480) -> (element=w489:dbl)
    n191 = Subtract(x=w478, y=w477) -> (x-y=w476:dbl)
    n192 = Subtract(x=w487, y=w489) -> (x-y=w486:dbl)
    n193 = Divide(x=w476, y=w475) -> (x/y=→"Vx (cm/s)":dbl)
    n194 = Divide(x=w486, y=w475) -> (x/y=→"Vy (cm/s)":dbl)
    n195 = Wait Until Next ms Multiple(millisecond multiple=u32 33) -> ()  [unwired: 1 out]
  }
  n196 = call <vilib>:"Space Constant.vi"() -> ("String"=w16:string)
  n197 = Format Into String("Dst") -> (resulting string=w17:string)  [unwired: 3 in, 1 out]
  n198 = Format Into String("Address") -> (resulting string=w19:string)  [unwired: 3 in, 1 out]
  n199 = Concatenate Strings("c0 " ("string"), w17, w16, w19, w16) -> (w6:string)
  n200 = flat-sequence {
    tunnel: [w506] -> w15
    tunnel: [w519] -> w14
    tunnel: [w518] -> w13
    tunnel: w11 -> [w517]
    tunnel: "stop bits" -> [w516]
    tunnel: "flow control" -> [w515]
    tunnel: "baud rate (115200)" -> [w514]
    tunnel: "data bits (8)" -> [w513]
    tunnel: "parity (0:none)" -> [w512]
    tunnel: w11 -> [w511]
    tunnel: "parity (0:none)" -> [w510]
    tunnel: "data bits (8)" -> [w509]
    tunnel: "stop bits" -> [w508]
    tunnel: "flow control" -> [w507]
    tunnel: w6 -> [w505]
    tunnel: w15 -> [w572]
    tunnel: w14 -> [w570]
    tunnel: w13 -> [w569]
    tunnel: [w571] -> w3
    tunnel: [w568] -> w2
    tunnel: [w567] -> w1
    tunnel: [w590] -> w4
    tunnel: [w589] -> w5
    tunnel: [w592] -> w22
    tunnel: w3 -> [w592]
    tunnel: w2 -> [w588]
    tunnel: w1 -> [w591]
    frame #0 {
      n201 = while {
        tunnel: [w535] -> w519
        tunnel: [w534] -> w518
        tunnel: w517 -> [w533]
        tunnel: w516 -> [w532]
        tunnel: w515 -> [w531]
        tunnel: w514 -> [w530]
        tunnel: w513 -> [w529]
        tunnel: w512 -> [w528]
        tunnel: w511 -> [w527]
        tunnel: w510 -> [w526]
        tunnel: w509 -> [w525]
        tunnel: w508 -> [w524]
        tunnel: w507 -> [w523]
        tunnel: [w522] -> w506
        tunnel: w505 -> [w521]
        stop <- "Reaction Wheel" stop-if-true
        n202 = case shown="True" "Reaction Wheel" {
          tunnel: [_ w554] -> w535
          tunnel: [_ w553] -> w534
          tunnel: w533 -> [_ w552]
          tunnel: w532 -> [_ w551]
          tunnel: w531 -> [_ w550]
          tunnel: w530 -> [_ w549]
          tunnel: w529 -> [_ w548]
          tunnel: w528 -> [_ w547]
          tunnel: w527 -> [_ w546]
          tunnel: w526 -> [_ w545]
          tunnel: w525 -> [_ w544]
          tunnel: w524 -> [_ w543]
          tunnel: w523 -> [_ w542]
          tunnel: [_ w541] -> w522
          tunnel: w521 -> [_ w538]
          frame False {
            n203 = Wait Until Next ms Multiple(millisecond multiple=u32 100) -> ()  [unwired: 1 out]
          }
          frame True {
            # "Perform a write operation on one serial port"
            # "Ping and Init"
            n204 = Concatenate Strings(w538, "a0 07 40 c0" ("string")) -> (w539:string)
            n205 = call-poly "VISA Configure Serial Port"("VISA resource name"="VISA resource name (write)", "timeout (10sec)"=w552, "baud rate (9600)"=w545, "data bits (8)"=w544, "stop bits (10: 1 bit)"=w551, "flow control (0:none)"=w550) -> ("VISA resource name out"=w555:refnum<visa-resource-name>, "error out"=w560:errorcluster)  [unwired: 3 in, 5 out]
            n206 = call-poly "VISA Configure Serial Port"("VISA resource name"="VISA resource name (write)", "timeout (10sec)"=w546, "baud rate (9600)"=w549, "data bits (8)"=w548, "parity (0:none)"=w547, "error in (no error)"=w560, "stop bits (10: 1 bit)"=w543, "flow control (0:none)"=w542) -> ("VISA resource name out"=w556:refnum<visa-resource-name>, "error out"=w561:errorcluster)  [unwired: 2 in, 4 out]
            n207 = VISA Write(VISA resource name=w555, write buffer=w539, error in (no error)=w561) -> (VISA resource name out=w563:refnum<visa-resource-name>, error out=w562:errorcluster)  [unwired: 1 out]
            n208 = VISA Read(VISA resource name=w556, byte count="bytes to read", error in (no error)=w562) -> (VISA resource name out=w541:refnum<visa-resource-name>, read buffer=→"Read string":string, return count=→"bytes read":u32, error out=w564:errorcluster)
            n209 = Concatenate Strings(w538, "a1 00 20 00 00 28 59 c0" ("string")) -> (w566:string)
            n210 = VISA Write(VISA resource name=w563, write buffer=w566, error in (no error)=w564) -> (VISA resource name out=w554:refnum<visa-resource-name>, error out=w553:errorcluster)  [unwired: 1 out]
          }
        }
      }
    }
    frame #1 {
      n211 = while {
        tunnel: w572 -> [w583]
        tunnel: [w583] -> w571
        tunnel: w570 -> [w582]
        tunnel: w569 -> [w581]
        tunnel: [w580] -> w568
        tunnel: [w579] -> w567
        stop <- w584 stop-if-true
        n212 = Wait Until Next ms Multiple(millisecond multiple=u32 25) -> ()  [unwired: 1 out]
        n213 = local read "Dst"() -> (w578:i32)
        n214 = call "CmdGenerate.vi"("Control Value"="Control Value", "Mode"="Control Mode", "Dst"=w578) -> ("CMD code"=w574:string)
        "Write String" <- w574
        n215 = VISA Write(VISA resource name=w582, write buffer=w574, error in (no error)=w581) -> (VISA resource name out=w579:refnum<visa-resource-name>, return count=→"bytes written":u32, error out=w580:errorcluster)
        n216 = local read "STOP"() -> (w584:bool)
      }
    }
    frame #2 {
      # "Set to Idle"
      n217 = local read "Dst"() -> (w587:i32)
      n218 = call "CmdGenerate.vi"("Mode"=0, "Dst"=w587) -> ("CMD code"=w585:string)  [unwired: 1 in]
      n219 = VISA Write(VISA resource name=w591, write buffer=w585, error in (no error)=w588) -> (VISA resource name out=w590:refnum<visa-resource-name>, error out=w589:errorcluster)  [unwired: 1 out]
    }
  }
  n220 = VISA Close(VISA resource name=w4, error in (no error)=w5) -> (error out=w24:errorcluster)
  n221 = VISA Close(VISA resource name=w22, error in (no error)=w24) -> (error out=w23:errorcluster)
  n222 = call <vilib>:"Simple Error Handler.vi"("error in (no error)"=w23) -> ()  [unwired: 1 in, 8 out]
  n223 = local write "STOP"(w40) -> ()
  n224 = VISA Close(VISA resource name=w33, error in (no error)=w32) -> ()  [unwired: 1 out]
  n225 = call <vilib>:"DAQmx Clear Task.vi"("task in"=w53, "error in"=w54) -> ("error out"=w59:errorcluster)  [unwired: 13 in]
  n226 = call <vilib>:"Simple Error Handler.vi"("type of dialog (OK msg:1)"=w60, "error in (no error)"=w59) -> ()  [unwired: 3 in, 5 out]
